vi "Stop.vi"(8 "error in (no error)":errorcluster, 11 "Electrophysiology in":refnum<class "IntanElectrophysiology.lvclass">) -> (0 "error out":errorcluster, 3 "Electrophysiology out":refnum<class "IntanElectrophysiology.lvclass">)   [LabVIEW 2014, in "IntanElectrophysiology.lvclass"]
uses:
  IntanElectrophysiology.lvclass
  IntanElectrophysiology.lvclass/IntanElectrophysiology.ctl
  AcquireTraces/AcquireTraces.lvclass/AcquireTraces.ctl
  HDF5Tools/LabView/HDF5Tools.lvlib
  AcquireTraces/AcquireTraces.lvclass
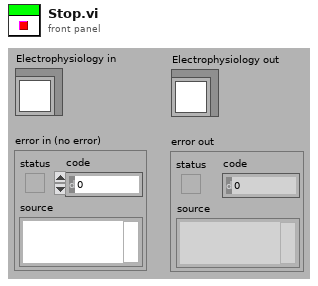
[diagram p1: front panel]
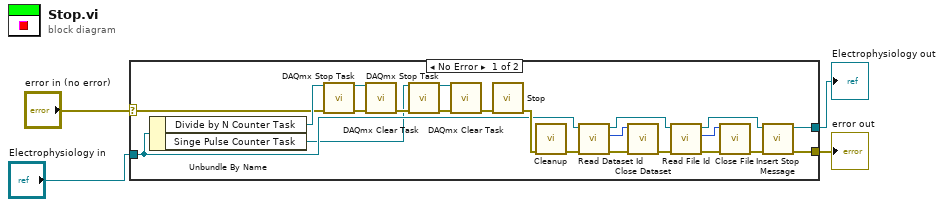
[diagram p0: block diagram]
diagram:
  n1 = case shown="No Error" "error in (no error)" {
    selector: "error in (no error)" -> [w10 w28]
    tunnel: [w25 w28] -> w2
    tunnel: [w24 w27] -> w4
    tunnel: "Electrophysiology in" -> [w14 w27]
    frame No Error {
      n2 = Unbundle By Name(w14) -> ("Divide by N Counter Task"=w11:refnum<k21>, "Singe Pulse Counter Task"=w7:refnum<k21>)
      n3 = call <vilib>:"DAQmx Stop Task.vi"("task/channels in"=w11, "error in"=w10) -> ("task out"=w13:refnum<k21>, "error out"=w12:errorcluster)  [unwired: 12 in]
      n4 = call <vilib>:"DAQmx Clear Task.vi"("task in"=w13, "error in"=w12) -> ("error out"=w9:errorcluster)  [unwired: 13 in]
      n5 = call <vilib>:"DAQmx Stop Task.vi"("task/channels in"=w7, "error in"=w9) -> ("task out"=w6:refnum<k21>, "error out"=w8:errorcluster)  [unwired: 12 in]
      n6 = call <vilib>:"DAQmx Clear Task.vi"("task in"=w6, "error in"=w8) -> ("error out"=w5:errorcluster)  [unwired: 13 in]
      n7 = call "Stop.vi"("error in (no error)"=w5) -> ("error out"=w19:errorcluster)  [unwired: 9 in, 1 out]
      n8 = call "Cleanup.vi"("error in (no error)"=w19) -> ("error out"=w18:errorcluster)  [unwired: 9 in, 1 out]
      n9 = call-dynamic "Read Dataset Id.vi"("error in (no error)"=w18, "AcquireTraces in"=w14) -> ("error out"=w17:errorcluster, "Dataset Id"=w23:u64, "AcquireTraces out"=w22:refnum<class "IntanElectrophysiology.lvclass">)  [unwired: 7 in]
      n10 = call "Close Dataset.vi"("error in (no error)"=w17, "dataset_id"=w23) -> ("error out"=w16:errorcluster)  [unwired: 9 in]
      n11 = call "Read File Id.vi"("error in (no error)"=w16, "AcquireTraces in"=w22) -> ("error out"=w15:errorcluster, "File Id"=w21:u64, "AcquireTraces out"=w20:refnum<class "IntanElectrophysiology.lvclass">)  [unwired: 7 in]
      n12 = call "Close File.vi"("error in (no error)"=w15, "file_id"=w21) -> ("error out"=w26:errorcluster)  [unwired: 9 in]
      n13 = call-dynamic "Insert Stop Message.vi"("error in (no error)"=w26, "Electrophysiology in"=w20) -> ("error out"=w25:errorcluster, "Electrophysiology out"=w24:refnum<class "IntanElectrophysiology.lvclass">)  [unwired: 8 in]
    }
    frame Error {
    }
  }
  "error out" <- w2
  "Electrophysiology out" <- w4
